vi "PS90_FreeSwitch.vi"(8 "error in (no error)":errorcluster, 9 "Axis number":i32=1 min=1 max=9, 10 "Control unit ID":i32=1 min=1 max=10, 11 "DLOwis.lvclass":refnum<class "DLOwis.lvclass">) -> (0 "error out":errorcluster, 3 "DLOwis.lvclass":refnum<class "DLOwis.lvclass">)   [LabVIEW 2019, in "DLOwis.lvclass"]
doc: "PS90_FreeSwitch.vi, created: 17.10.2006 alex; last change: 19.07.2016 alex;\n\n<B>FUNCTION:</B> \n\nRelease active limit switches of an axis.\nAfter an axis has driven into a limit switch, it can release a limit switch with\nthis function. This is valid only for released axes. Besides, the direction of\nthe movement is selected automatically, depending on whether a positive\nor negative limit switch is activated.\n----------------------------------------------------------------------------------------\n<B>INPUT:</B>\n[I32] <B>Control unit ID:</B> control unit index. (Default=1, Range=1...10) \n[I32] <B>Axis number:</B> axis number. (Default=1, Range=1...9) \n[CLU] <B>error in</B>\n----------------------------------------------------------------------------------------\n<B>OUTPUT:</B>\n[CLU] <B>error out</B>\n----------------------------------------------------------------------------------------\n<B>SUB-VIs:</B>\n----------------------------------------------------------------------------------------\n<B>EXT-Calls:</B>\nps90.dll (V2.00)\n----------------------------------------------------------------------------------------"
uses:
  DLOwis.lvclass
  C:/Users/elysium/Documents/dev/TRANCON/Classes/Delay Line/DelayLine.lvclass
  DelayLine.lvclass/DelayLine.ctl
  DelayLine.lvclass
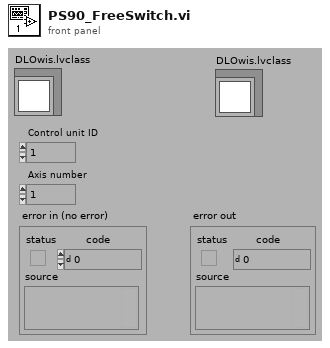
[diagram p1: front panel]
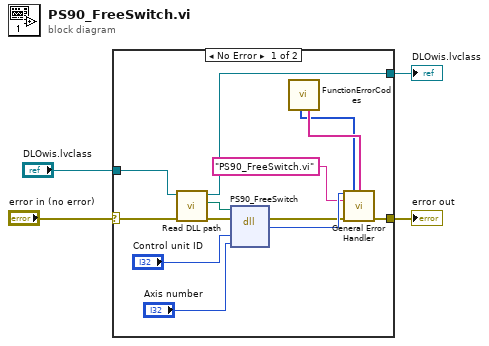
[diagram p0: block diagram]
diagram:
  n1 = case shown="No Error" "error in (no error)" {
    selector: "error in (no error)" -> [w7 w19]
    tunnel: [w16 w19] -> w4
    tunnel: "DLOwis.lvclass" -> [w10 w18]
    tunnel: [w5 w18] -> w1
    frame No Error {
      n2 = call "Read DLL path.vi"("error in (no error)"=w7, "DelayLine in"=w10) -> ("error out"=w8:errorcluster, "DLL path"=w9:path, "DelayLine out"=w5:refnum<class "DLOwis.lvclass">)  [unwired: 7 in]
      n3 = dll-call lib="C:/Users/Sergey Denisov/Documents/REPS/TRANCON/DLL/ps90.dll" fn="PS90_FreeSwitch"(path in=w9, error in=w8, "Index"="Control unit ID", "AxisNr"="Axis number") -> (error out=w6:errorcluster, "Rückgabetyp"=w15:i32)  [unwired: 3 in, 1 out]
      n4 = call "FunctionErrorCodes.vi"() -> ("[user-defined codes]"=w11:i32[], "[user-defined descriptions]"=w12:string[])  [unwired: 8 in]
      n5 = call <vilib>:"General Error Handler.vi"("[error code] (0)"=w15, "[user-defined codes]"=w11, "[user-defined descriptions]"=w12, "[error source] (\" \")"="PS90_FreeSwitch.vi" ("[error source] (\" \")"), "error in (no error)"=w6) -> ("error out"=w16:errorcluster)  [unwired: 6 in, 4 out]
    }
    frame Error {
    }
  }
  "error out" <- w4
  "DLOwis.lvclass" <- w1
